vi "Telegram-Example.vi"() -> ()   [LabVIEW 2015]
doc: "Created IvanLis by LabVIEW Portal\nProfile: http://labviewportal.org/memberlist.php?mode=viewprofile&u=987\neMail: IvanLisanov@gMail.com\nTelegram: https://t.me/IvanLis"
uses:
  TypeDef/Client Command TypeDef.ctl
  TypeDef/Command Enum TypeDef.ctl
  Telegram Library/Telegram Class/Telegram Class.lvclass
  <vilib>/event_ctls.llb/usereventprio.ctl
  JSON Library/TypeDef/Message Text Out.ctl
  Telegram Library/TypeDef/TDLib Parameters.ctl
  JSON Library/JSON Library.lvlib
  Telegram Library/Telegram Library.lvlib
panel:
  in  "Message's":string
  in  "Message Out":string
  in  "Tab Control":enum32{"Chat's", "User's"}(tab)
  in  "Chat's":i32(listbox)
  in  "User's":i32(listbox)
  in  "Send Message":bool
  out "ConnectionState":string
  out "JSON":string
  out "Client ID":i32
  out "error":errorcluster
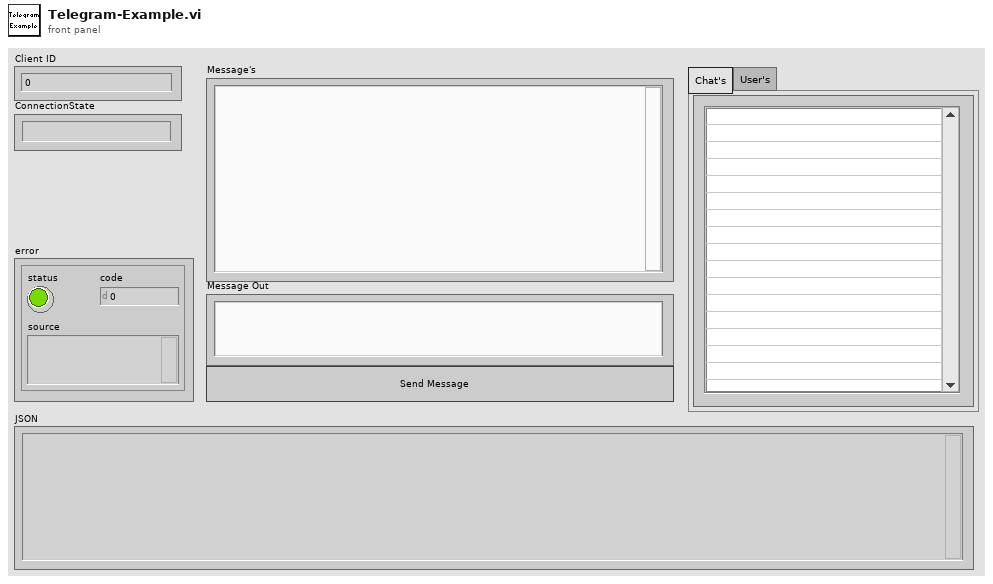
[diagram p1: front panel]
types:
  T1 = typedef "Client Command TypeDef.ctl" = cluster{"Command":T2, "Data":variant}
  T2 = typedef "Command Enum TypeDef.ctl" = enum16{"empty", "ClearControl", "Client Initialize", "Client Destroy", "Client Create", "Log Verbosity", "Test Execute", "Client Start", "Client Receive", "send_setTdlibParameters", "send_checkDatabaseEncryptionKey", "send_authorizationStateWaitPhoneNumber", "send_authorizationStateWaitCode", "send_getChats", "send_getChatHistory", "connectionState", "SendMessage", "Select Chat", "Select User"}
  T3 = typedef "usereventprio.ctl" = enum32{"high priority", "normal priority"}
  T4 = cluster{"@type":string, "new_verbosity_level":i32}
  T5 = cluster{"@type":string, "text":string, "@extra":string}
  T6 = typedef "JSON Library.lvlib/Message Text Out.ctl" = cluster{"@type":string, "chat_id":i64, "input_message_content":cluster{"@type":string, "text":cluster{"@type":string, "text":string}}}
  T7 = typedef "Telegram Library.lvlib/TDLib Parameters.ctl" = cluster{"database_directory":string, "use_file_database":bool, "use_chat_info_database":bool, "use_message_database":bool, "use_secret_chats":bool, "api_id":i32, "api_hash":string, "system_language_code":string, "device_model":string, "application_version":string, "enable_storage_optimizer":bool}
  T8 = cluster{"@type":string, "chat_id":i64, "from_message_id":i64, "limit":i32, "onlyLocal":bool}
  T9 = typedef "Telegram Library.lvlib/Telegram State.ctl" = enum16{"empty", "ok", "authorizationStateClosed", "authorizationStateWaitTdlibParameters", "authorizationStateWaitEncryptionKey", "authorizationStateWaitPhoneNumber", "authorizationStateWaitCode", "connectionStateWaitingForNetwork", "connectionStateConnectingToProxy", "connectionStateUpdating", "connectionStateConnecting", "connectionStateReady", "updateUser_user", "updateNewChat_chat", "updateNewMessage_Text", "updateChatLastMessage_Text", "updateDeleteMessages", "updateChatPosition", "ChatHistoryMessages_Text"}
  T10 = typedef "Telegram Library.lvlib/Chat.ctl" = cluster{"id":i64, "position":i64, "title":string}
  T11 = typedef "Telegram Library.lvlib/User.ctl" = cluster{"id":i64, "phone_number":string, "username":string, "last_name":string, "first_name":string}
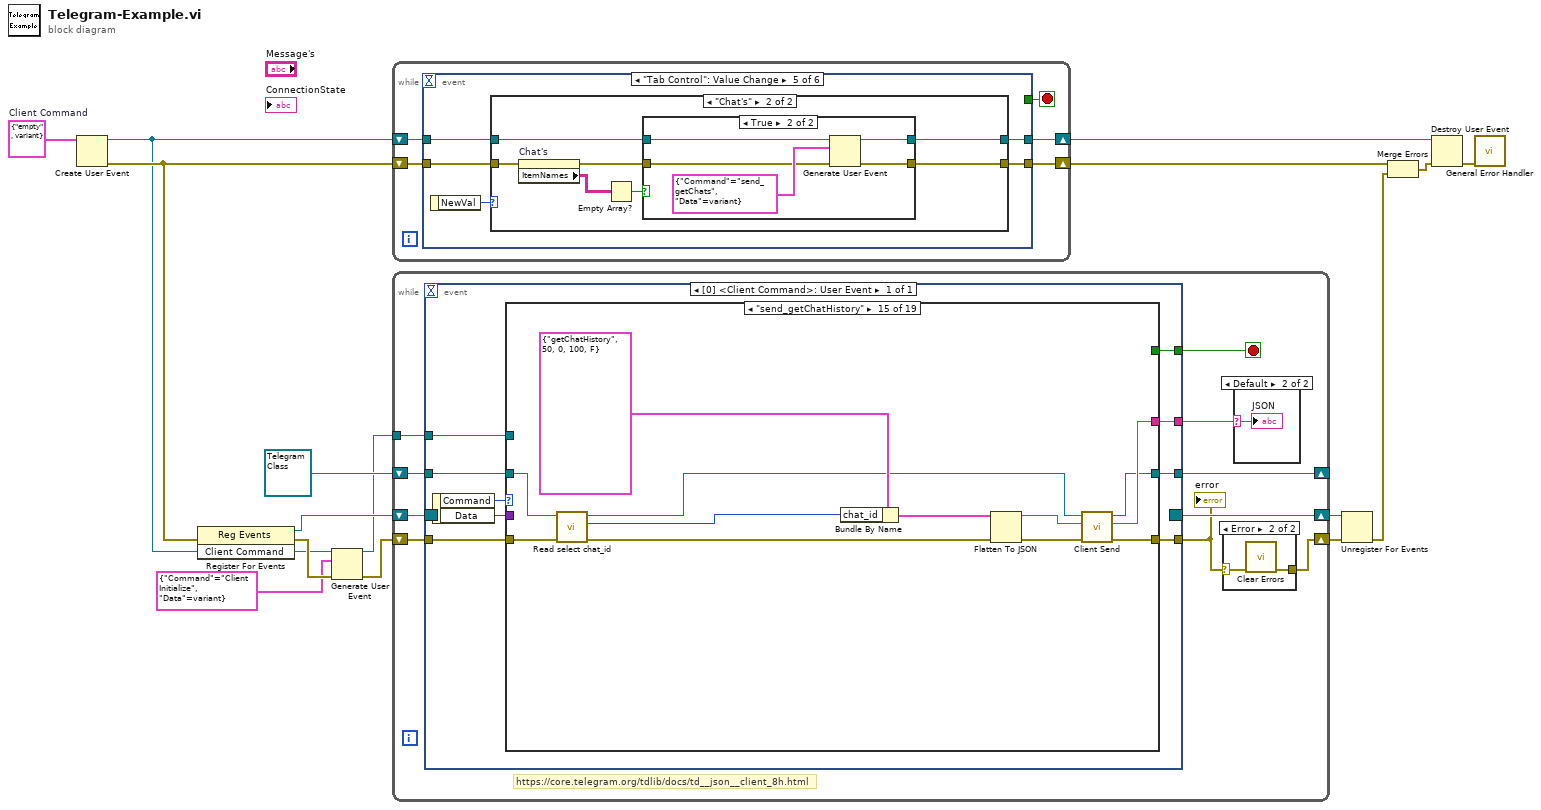
[diagram p0: block diagram]
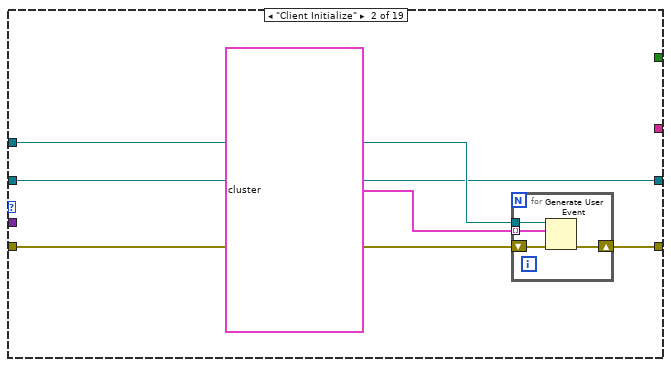
[diagram p5: hidden frame]
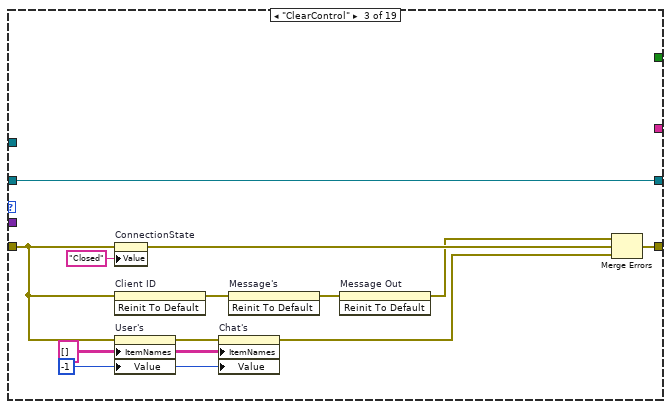
[diagram p6: hidden frame]
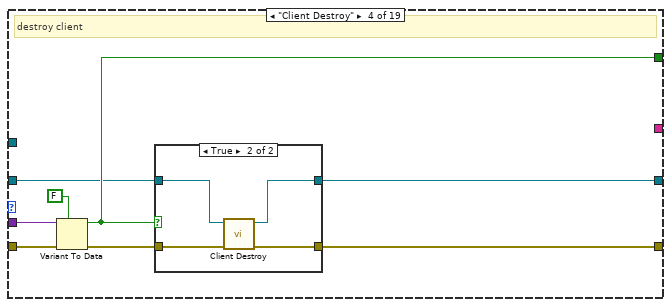
[diagram p7: hidden frame]
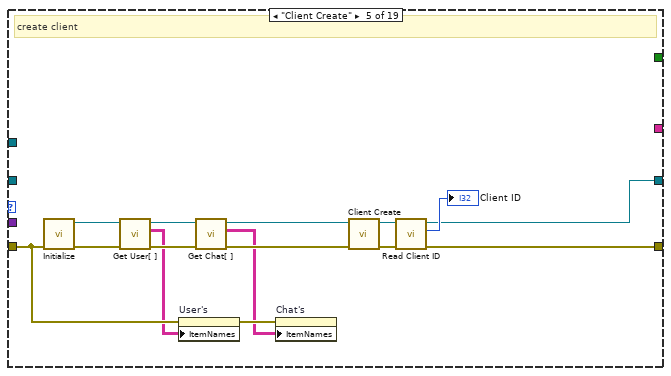
[diagram p9: hidden frame]
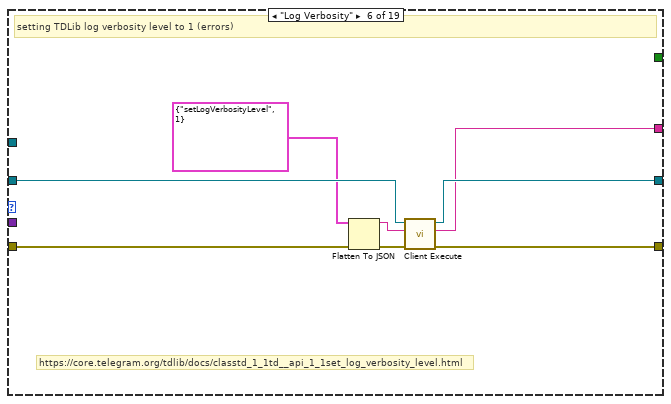
[diagram p10: hidden frame]
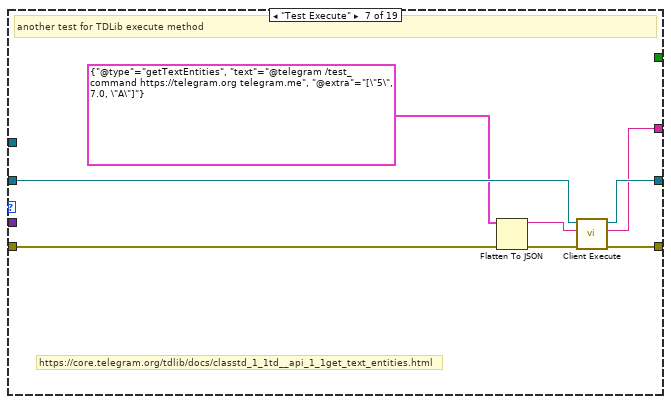
[diagram p11: hidden frame]
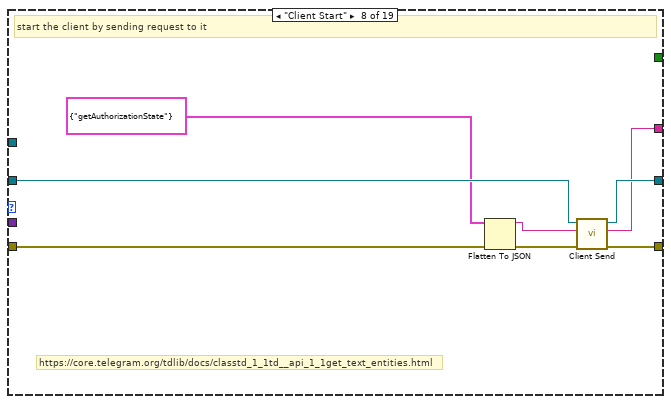
[diagram p12: hidden frame]
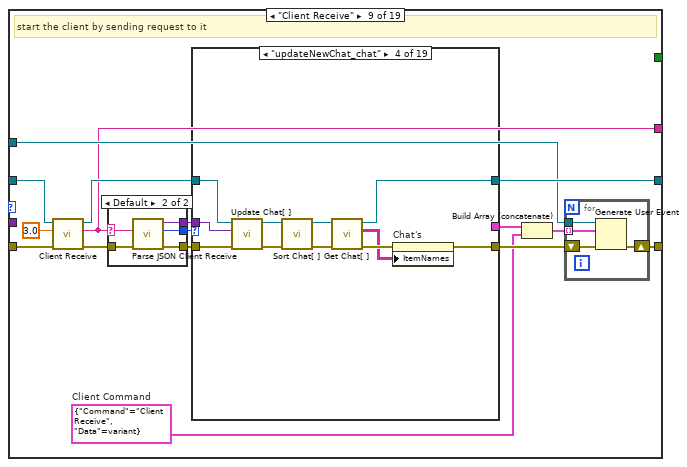
[diagram p13: hidden frame]
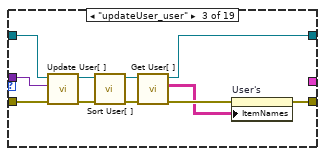
[diagram p17: hidden frame]
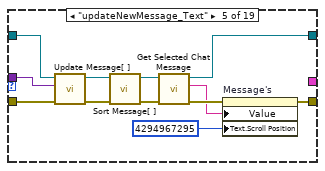
[diagram p18: hidden frame]
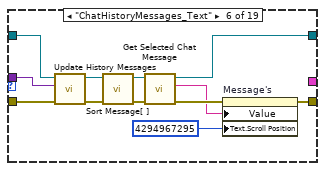
[diagram p19: hidden frame]
diagram:
  w15 = T1 {"Command"=enum."empty", "Data"=variant}  # Client Command
  n1 = Create User Event(user event datatype=w15) -> (user event=w3:refnum<user-event>, error out=w14:errorcluster)  [unwired: 1 in]
  n2 = register-events(error in=w14, w3) -> (reference out=w13:refnum<event-registration>, error out=w5:errorcluster)  [unwired: 1 in]
  n3 = Generate User Event(user event=w3, event data cluster=T1 {"Command"=enum."Client Initialize", "Data"=variant} ("event data"), error in=w5) -> (user event out=w2:refnum<user-event>, error out=w6:errorcluster)  [unwired: 1 in]
  n4 = while {
    shift-right: [w18] -> w10
    shift-left: w3 -> [w20]
    shift-right: [w17] -> w16
    shift-left: w14 -> [w19]
    stop <- w21 stop-if-true
    n5 = event shown="[4] \"Tab Control\": Value Change" {
      selector: _ -> [_ _ _ _ _ _]
      dyn-events: _ -> [_ _ _ _ _ _]
      timeout: _ -> [_ _ _ _ _ _]
      tunnel: [_ _ _ _ _ w71] -> w21
      tunnel: w20 -> [w26 w33 w40 w45 w50 w76]
      tunnel: w19 -> [w25 w32 w39 w44 w49 w75]
      tunnel: [w28 w35 w42 w47 w52 w78] -> w18
      tunnel: [w27 w34 w41 w46 w51 w77] -> w17
      event "Send Message": Value Change {
        n6 = event-data() -> ()  [unwired: 1 in, 1 out]
        n7 = Bundle By Name(cluster=T1 {"Command"=enum."SendMessage", "Data"=variant} ("event data"), "Data"="Message Out") -> (w23:T1)
        n8 = Generate User Event(user event=w26, event data cluster=w23, error in=w25) -> (user event out=w28:refnum<user-event>, error out=w27:errorcluster)  [unwired: 1 in]
      }
      event "Chat's": Value Change {
        n9 = event-data() -> ("NewVal"=w29:i32)  [unwired: 1 in]
        n10 = Bundle By Name(cluster=T1 {"Command"=enum."Select Chat", "Data"=variant} ("event data"), "Data"=w29) -> (w30:T1)
        n11 = Generate User Event(user event=w33, event data cluster=w30, error in=w32) -> (user event out=w35:refnum<user-event>, error out=w34:errorcluster)  [unwired: 1 in]
      }
      event "User's": Value Change {
        n12 = event-data() -> ("NewVal"=w36:i32)  [unwired: 1 in]
        n13 = Bundle By Name(cluster=T1 {"Command"=enum."Select User", "Data"=variant} ("event data"), "Data"=w36) -> (w37:T1)
        n14 = Generate User Event(user event=w40, event data cluster=w37, error in=w39) -> (user event out=w42:refnum<user-event>, error out=w41:errorcluster)  [unwired: 1 in]
      }
      event "Chat's": Double Click {
        n15 = event-data() -> ()  [unwired: 1 in, 4 out]
        n16 = Generate User Event(user event=w45, event data cluster=T1 {"Command"=enum."send_getChatHistory", "Data"=variant} ("event data"), error in=w44) -> (user event out=w47:refnum<user-event>, error out=w46:errorcluster)  [unwired: 1 in]
      }
      event "Tab Control": Value Change {
        n17 = event-data() -> ("NewVal"=w48:enum32{"Chat's", "User's"})  [unwired: 1 in]
        n18 = case shown="\"Chat's\"" w48 {
          tunnel: [w54 w61] -> w52
          tunnel: [w53 w60] -> w51
          tunnel: w50 -> [w54 w59]
          tunnel: w49 -> [w53 w58]
          frame Default {
          }
          frame "Chat's" {
            n19 = property on="Chat's" class="MCListbox (strict)"(error in=w58) -> (error out=w57:errorcluster, "ItemNames"=w56:string[][])  [unwired: 1 in, 1 out]
            n20 = Empty Array?(array=w56) -> (empty?=w55:bool)
            n21 = case shown="True" w55 {
              tunnel: [w63 w68] -> w61
              tunnel: [w62 w67] -> w60
              tunnel: w59 -> [w63 w66]
              tunnel: w57 -> [w62 w64]
              frame False {
              }
              frame True {
                n22 = Generate User Event(user event=w66, event data cluster=T1 {"Command"=enum."send_getChats", "Data"=variant} ("event data"), error in=w64) -> (user event out=w68:refnum<user-event>, error out=w67:errorcluster)  [unwired: 1 in]
              }
            }
          }
        }
      }
      event Panel Close? {
        w71 = TRUE
        n23 = event-data() -> ()  [unwired: 1 in, 1 out]
        n24 = Bundle By Name(cluster=T1 {"Command"=enum."Client Destroy", "Data"=variant} ("event data"), "Data"=w71) -> (w72:T1)
        n25 = Build Array(T1 {"Command"=enum."ClearControl", "Data"=variant} ("event data"), w72) -> (w70:T1[])
        n26 = for {
          tunnel: usereventprio."high priority" ("priority (normal)") -> [w80]
          tunnel: w70 -> [w79] mode=indexing
          shift-right: [w84] -> w78
          shift-left: w76 -> [w82]
          shift-right: [w83] -> w77
          shift-left: w75 -> [w81]
          n27 = Generate User Event(priority (normal)=w80, user event=w82, event data cluster=w79, error in=w81) -> (user event out=w84:refnum<user-event>, error out=w83:errorcluster)
        }
        n28 = event-data("Discard?"=w71) -> ()  [unwired: 1 in, 1 out]
      }
    }
  }
  n29 = while {
    shift-right: [w91] -> w12
    shift-left: w13 -> [w93]
    shift-right: [w85] -> w11
    shift-left: w6 -> [w92]
    tunnel: w2 -> [w88]
    shift-right: [w90] -> _
    shift-left: refnum<class "Telegram Class.lvclass"> refnum ("Telegram Class out") -> [w89]
    stop <- w94 stop-if-true
    # "https://core.telegram.org/tdlib/docs/td__json__client_8h.html"
    n30 = event shown="[0] <Client Command>: User Event" {
      selector: w93 -> [_]
      dyn-events: [_] -> w91
      timeout: _ -> [_]
      tunnel: [w103] -> w94
      tunnel: w92 -> [w107]
      tunnel: [w104] -> w86
      tunnel: [w102] -> w90
      tunnel: w89 -> [w101]
      tunnel: [w100] -> w87
      tunnel: w88 -> [w99]
      event User Event {
        n31 = event-data() -> ("Command"=w106:T2, "Data"=w105:variant)  [unwired: 1 in]
        n32 = case shown="\"send_getChatHistory\"" w106 {
          tunnel: w107 -> [w109 w110 w123 w138 w147 w162 w170 w177 w199 w336 w360 w370 w378 w386 w397 w409 w419 w456 w471]
          tunnel: w105 -> [_ _ _ w137 _ _ _ _ _ w335 w361 _ _ _ _ _ _ w455 w470]
          tunnel: [w109 w114 w122 w133 w149 w167 w175 w183 w190 w345 w362 w375 w383 w391 w403 w415 w424 w439 w472] -> w104
          tunnel: [_ _ _ w135 _ _ _ _ _ _ _ _ _ _ _ _ _ _ _] -> w103
          tunnel: [w108 w111 w127 w132 w150 w165 w173 w181 w193 w346 w363 w373 w381 w389 w401 w413 w422 w444 w473] -> w102
          tunnel: w101 -> [w108 w111 w127 w131 _ w166 w174 w182 w198 w340 w363 w369 w376 w384 w396 w405 w420 w457 w474]
          tunnel: [_ _ _ _ _ w164 w172 w180 w187 w344 _ w374 w382 w390 w402 w414 w423 _ _] -> w100
          tunnel: w99 -> [_ w113 _ _ _ _ _ _ w188 _ _ _ _ _ _ _ _ w438 _]
          frame "empty" {
          }
          frame "Client Initialize" {
            n33 = for {
              shift-right: [w117] -> w114
              shift-left: w110 -> [w118]
              tunnel: w113 -> [w116]
              tunnel: T1[] [{"Command"=enum."ClearControl", "Data"=variant}, {"Command"=enum."Client Create", "Data"=variant}, {"Command"=enum."Log Verbosity", "Data"=variant}, {"Command"=enum."Test Execute", "Data"=variant}, {"Command"=enum."Client Start", "Data"=variant}, {"Command"=enum."Client Receive", "Data"=variant}] -> [w115] mode=indexing
              n34 = Generate User Event(user event=w116, event data cluster=w115, error in=w118) -> (error out=w117:errorcluster)  [unwired: 1 in, 1 out]
            }
          }
          frame "ClearControl" {
            w126 = string[][] [] ("Item Names")
            w129 = -1 ("Focus Row")
            n35 = property on="ConnectionState" class="Str"(error in=w123, "Value"="Closed" ("ConnectionState")) -> (error out=w121:errorcluster)  [unwired: 1 in, 1 out]
            n36 = invoke on="Client ID" class="DigNum (strict)" method="Reinit To Default"(error in=w123) -> (error out=w124:errorcluster)  [unwired: 2 in, 2 out]
            n37 = property on="User's" class="MCListbox (strict)"(error in=w123, "ItemNames"=w126, "Value"=w129) -> (error out=w128:errorcluster)  [unwired: 1 in, 1 out]
            n38 = property on="Chat's" class="MCListbox (strict)"(error in=w128, "ItemNames"=w126, "Value"=w129) -> (error out=w119:errorcluster)  [unwired: 1 in, 1 out]
            n39 = invoke on="Message's" class="Str" method="Reinit To Default"(error in=w124) -> (error out=w125:errorcluster)  [unwired: 2 in, 2 out]
            n40 = invoke on="Message Out" class="Str" method="Reinit To Default"(error in=w125) -> (error out=w120:errorcluster)  [unwired: 2 in, 2 out]
            n41 = Merge Errors(w120, w121, w119) -> (w122:errorcluster)
          }
          frame "Client Destroy" {
            # "destroy client"
            n42 = Variant To Data(error in=w138, type=FALSE, Variant=w137) -> (data=w135:bool, error out=w134:errorcluster)
            n43 = case shown="True" w135 {
              tunnel: w134 -> [w139 w144]
              tunnel: [w139 w141] -> w133
              tunnel: [w140 w142] -> w132
              tunnel: w131 -> [w140 w143]
              frame False {
              }
              frame True {
                n44 = call-dynamic "Client Destroy.vi"("error in (no error)"=w144, "Telegram Class in"=w143) -> ("error out"=w141:errorcluster, "Telegram Class out"=w142:refnum<class "Telegram Class.lvclass">)  [unwired: 8 in]
              }
            }
          }
          frame "Client Create" {
            # "create client"
            n45 = call "Initialize.vi"("error in (no error)"=w147) -> ("error out"=w154:errorcluster, "Telegram Class out"=w155:refnum<class "Telegram Class.lvclass">)  [unwired: 9 in]
            n46 = call-dynamic "Get User[ ].vi"("error in (no error)"=w154, "Telegram Class in"=w155) -> ("error out"=w153:errorcluster, "User[ ]"=w146:string[][], "Telegram Class out"=w156:refnum<class "Telegram Class.lvclass">)  [unwired: 7 in]
            n47 = property on="User's" class="MCListbox (strict)"(error in=w147, "ItemNames"=w146) -> (error out=w148:errorcluster)  [unwired: 1 in, 1 out]
            n48 = call-dynamic "Get Chat[ ].vi"("error in (no error)"=w153, "Telegram Class in"=w156) -> ("error out"=w152:errorcluster, "Chat[ ]"=w145:string[][], "Telegram Class out"=w151:refnum<class "Telegram Class.lvclass">)  [unwired: 7 in]
            n49 = property on="Chat's" class="MCListbox (strict)"(error in=w148, "ItemNames"=w145) -> ()  [unwired: 1 in, 2 out]
            n50 = call-dynamic "Client Create.vi"("error in (no error)"=w152, "Telegram Class in"=w151) -> ("error out"=w159:errorcluster, "Telegram Class out"=w158:refnum<class "Telegram Class.lvclass">)  [unwired: 8 in]
            n51 = call-dynamic "Read Client ID.vi"("error in (no error)"=w159, "Telegram Class in"=w158) -> ("error out"=w149:errorcluster, "Client ID"=→"Client ID":i32, "Telegram Class out"=w150:refnum<class "Telegram Class.lvclass">)  [unwired: 7 in]
          }
          frame "Log Verbosity" {
            # "https://core.telegram.org/tdlib/docs/classtd_1_1td__api_1_1set_log_verbosity_level.html"
            # "setting TDLib log verbosity level to 1 (errors)"
            n52 = Flatten To JSON(anything=T4 {"@type"="setLogVerbosityLevel", "new_verbosity_level"=1}, error in (no error)=w162) -> (JSON string=w161:string, 11:w163:errorcluster)  [unwired: 1 in]
            n53 = call-dynamic "Client Execute.vi"("error in (no error)"=w163, "JSON (UTF-8) String In"=w161, "Telegram Class in"=w166) -> ("error out"=w167:errorcluster, "UTF-8 String Out"=w164:string, "Telegram Class out"=w165:refnum<class "Telegram Class.lvclass">)  [unwired: 6 in]
          }
          frame "Test Execute" {
            # "https://core.telegram.org/tdlib/docs/classtd_1_1td__api_1_1get_text_entities.html"
            # "another test for TDLib execute method"
            n54 = Flatten To JSON(anything=T5 {"@type"="getTextEntities", "text"="@telegram /test_command https://telegram.org telegram.me", "@extra"="[\"5\", 7.0, \"A\"]"}, error in (no error)=w170) -> (JSON string=w169:string, 11:w171:errorcluster)  [unwired: 1 in]
            n55 = call-dynamic "Client Execute.vi"("error in (no error)"=w171, "JSON (UTF-8) String In"=w169, "Telegram Class in"=w174) -> ("error out"=w175:errorcluster, "UTF-8 String Out"=w172:string, "Telegram Class out"=w173:refnum<class "Telegram Class.lvclass">)  [unwired: 6 in]
          }
          frame "Client Start" {
            # "https://core.telegram.org/tdlib/docs/classtd_1_1td__api_1_1get_text_entities.html"
            # "start the client by sending request to it"
            n56 = Flatten To JSON(anything=cluster{"@type":string} {"@type"="getAuthorizationState"} ("Message"), error in (no error)=w177) -> (JSON string=w179:string, 11:w178:errorcluster)  [unwired: 1 in]
            n57 = call-dynamic "Client Send.vi"("error in (no error)"=w178, "JSON (UTF-8) String In"=w179, "Telegram Class in"=w182) -> ("error out"=w183:errorcluster, "UTF-8 String Out"=w180:string, "Telegram Class out"=w181:refnum<class "Telegram Class.lvclass">)  [unwired: 6 in]
          }
          frame "Client Receive" {
            w184 = T1 {"Command"=enum."Client Receive", "Data"=variant}  # Client Command
            # "start the client by sending request to it"
            n58 = call-dynamic "Client Receive.vi"("error in (no error)"=w199, "Timeout"=3.0, "Telegram Class in"=w198) -> ("error out"=w196:errorcluster, "UTF-8 String Out"=w187:string, "Telegram Class out"=w192:refnum<class "Telegram Class.lvclass">)  [unwired: 6 in]
            n59 = case shown="Default" w187 {
              selector: w187 -> [_ w202]
              tunnel: w196 -> [w200 w205]
              tunnel: [_ w204] -> w195
              tunnel: [w200 w203] -> w194
              tunnel: [_ w201] -> w186
              frame "" {
              }
              frame Default {
                n60 = call "Parse JSON Client Receive.vi"("error in (no error)"=w205, "JSON (UTF-8) String"=w202) -> ("error out"=w203:errorcluster, "Telegram State"=w204:T9, "Message"=w201:variant)  [unwired: 7 in]
              }
            }
            n61 = case shown="\"updateNewChat_chat\"" w195 {
              tunnel: w194 -> [w210 w212 w224 w235 w247 w259 w260 w272 w277 w283 w286 w289 w292 w295 w301 w307 w313 w319 w326]
              tunnel: [w211 w213 w220 w231 w243 w255 w261 w267 w274 w284 w287 w290 w293 w296 w302 w308 w314 w320 w327] -> w193
              tunnel: w192 -> [w211 w213 w223 w234 w246 w258 w261 w271 w275 w284 w287 w290 w293 w296 w302 w308 w314 w320 w327]
              tunnel: [w210 w212 w221 w232 w244 w256 w260 w266 w276 w283 w286 w289 w292 w295 w301 w307 w313 w319 w326] -> w191
              tunnel: [_ _ _ _ _ _ _ _ _ w281 w285 w288 w291 w294 w299 w305 w311 w317 w324] -> w189
              tunnel: w186 -> [_ _ w222 w233 w245 w257 _ w270 w273 _ _ _ _ _ _ _ _ _ _]
              frame "empty" {
              }
              frame "ok" {
              }
              frame "updateUser_user" {
                n62 = call-dynamic "Update User[ ].vi"("error in (no error)"=w224, "Message"=w222, "Telegram Class in"=w223) -> ("error out"=w216:errorcluster, "Telegram Class out"=w217:refnum<class "Telegram Class.lvclass">)  [unwired: 7 in]
                n63 = call-dynamic "Sort User[ ].vi"("error in (no error)"=w216, "Telegram Class in"=w217) -> ("error out"=w214:errorcluster, "Telegram Class out"=w215:refnum<class "Telegram Class.lvclass">)  [unwired: 8 in]
                n64 = call-dynamic "Get User[ ].vi"("error in (no error)"=w214, "Telegram Class in"=w215) -> ("error out"=w219:errorcluster, "User[ ]"=w218:string[][], "Telegram Class out"=w220:refnum<class "Telegram Class.lvclass">)  [unwired: 7 in]
                n65 = property on="User's" class="MCListbox (strict)"(error in=w219, "ItemNames"=w218) -> (error out=w221:errorcluster)  [unwired: 1 in, 1 out]
              }
              frame "updateNewChat_chat" {
                n66 = call-dynamic "Update Chat[ ].vi"("error in (no error)"=w235, "Message"=w233, "Telegram Class in"=w234) -> ("error out"=w228:errorcluster, "Telegram Class out"=w225:refnum<class "Telegram Class.lvclass">)  [unwired: 7 in]
                n67 = call-dynamic "Sort Chat[ ].vi"("error in (no error)"=w228, "Telegram Class in"=w225) -> ("error out"=w227:errorcluster, "Telegram Class out"=w226:refnum<class "Telegram Class.lvclass">)  [unwired: 8 in]
                n68 = call-dynamic "Get Chat[ ].vi"("error in (no error)"=w227, "Telegram Class in"=w226) -> ("error out"=w230:errorcluster, "Chat[ ]"=w229:string[][], "Telegram Class out"=w231:refnum<class "Telegram Class.lvclass">)  [unwired: 7 in]
                n69 = property on="Chat's" class="MCListbox (strict)"(error in=w230, "ItemNames"=w229) -> (error out=w232:errorcluster)  [unwired: 1 in, 1 out]
              }
              frame "updateNewMessage_Text" {
                n70 = call-dynamic "Update Message[ ].vi"("error in (no error)"=w247, "Message"=w245, "Telegram Class in"=w246) -> ("error out"=w238:errorcluster, "Telegram Class out"=w239:refnum<class "Telegram Class.lvclass">)  [unwired: 7 in]
                n71 = call-dynamic "Sort Message[ ].vi"("error in (no error)"=w238, "Telegram Class in"=w239) -> ("error out"=w236:errorcluster, "Telegram Class out"=w237:refnum<class "Telegram Class.lvclass">)  [unwired: 8 in]
                n72 = call-dynamic "Get Selected Chat Message.vi"("error in (no error)"=w236, "Telegram Class in"=w237) -> ("error out"=w242:errorcluster, "Message's"=w241:string, "Telegram Class out"=w243:refnum<class "Telegram Class.lvclass">)  [unwired: 7 in]
                n73 = property on="Message's" class="Str"(error in=w242, "Value"=w241, "Text.Scroll Position"=u32 4294967295) -> (error out=w244:errorcluster)  [unwired: 1 in, 1 out]
              }
              frame "ChatHistoryMessages_Text" {
                n74 = call-dynamic "Update History Messages.vi"("error in (no error)"=w259, "Message"=w257, "Telegram Class in"=w258) -> ("error out"=w248:errorcluster, "Telegram Class out"=w251:refnum<class "Telegram Class.lvclass">)  [unwired: 7 in]
                n75 = call-dynamic "Sort Message[ ].vi"("error in (no error)"=w248, "Telegram Class in"=w251) -> ("error out"=w249:errorcluster, "Telegram Class out"=w250:refnum<class "Telegram Class.lvclass">)  [unwired: 8 in]
                n76 = call-dynamic "Get Selected Chat Message.vi"("error in (no error)"=w249, "Telegram Class in"=w250) -> ("error out"=w254:errorcluster, "Message's"=w253:string, "Telegram Class out"=w255:refnum<class "Telegram Class.lvclass">)  [unwired: 7 in]
                n77 = property on="Message's" class="Str"(error in=w254, "Value"=w253, "Text.Scroll Position"=u32 4294967295) -> (error out=w256:errorcluster)  [unwired: 1 in, 1 out]
              }
              frame "updateChatLastMessage_Text" {
              }
              frame "updateChatPosition" {
                n78 = call-dynamic "Update Chat Position.vi"("error in (no error)"=w272, "Message"=w270, "Telegram Class in"=w271) -> ("error out"=w265:errorcluster, "Telegram Class out"=w269:refnum<class "Telegram Class.lvclass">)  [unwired: 7 in]
                n79 = call-dynamic "Sort Chat[ ].vi"("error in (no error)"=w265, "Telegram Class in"=w269) -> ("error out"=w264:errorcluster, "Telegram Class out"=w268:refnum<class "Telegram Class.lvclass">)  [unwired: 8 in]
                n80 = call-dynamic "Get Chat[ ].vi"("error in (no error)"=w264, "Telegram Class in"=w268) -> ("error out"=w263:errorcluster, "Chat[ ]"=w262:string[][], "Telegram Class out"=w267:refnum<class "Telegram Class.lvclass">)  [unwired: 7 in]
                n81 = property on="Chat's" class="MCListbox (strict)"(error in=w263, "ItemNames"=w262) -> (error out=w266:errorcluster)  [unwired: 1 in, 1 out]
              }
              frame "updateDeleteMessages" {
                n82 = call-dynamic "Delete Messages.vi"("error in (no error)"=w277, "Message"=w273, "Telegram Class in"=w275) -> ("error out"=w276:errorcluster, "Telegram Class out"=w274:refnum<class "Telegram Class.lvclass">)  [unwired: 7 in]
              }
              frame "authorizationStateClosed" {
                # "if client is closed, we need to destroy it and create new client"
                n83 = Bundle By Name(cluster=T1 {"Command"=enum."connectionState", "Data"=variant} ("event data"), "Data"="Closed") -> (w279:T1)
                n84 = Build Array (concatenate)(w279, T1[] [{"Command"=enum."Client Destroy", "Data"=variant}, {"Command"=enum."Client Create", "Data"=variant}, {"Command"=enum."Log Verbosity", "Data"=variant}, {"Command"=enum."Test Execute", "Data"=variant}, {"Command"=enum."Client Start", "Data"=variant}]) -> (w281:T1[])
              }
              frame "authorizationStateWaitTdlibParameters" {
                w285 = T1[] [{"Command"=enum."send_setTdlibParameters", "Data"=variant}]  # Client Command's
                # "set TDLib parameters\nyou MUST obtain your own api_id and api_hash at \nhttps://my.telegram.org\nand use them in the setTdlibParameters call"
              }
              frame "authorizationStateWaitEncryptionKey" {
                w288 = T1[] [{"Command"=enum."send_checkDatabaseEncryptionKey", "Data"=variant}]  # Client Command's
                # "set an encryption key for database to let know TDLib how to open the database"
              }
              frame "authorizationStateWaitPhoneNumber" {
                w291 = T1[] [{"Command"=enum."send_authorizationStateWaitPhoneNumber", "Data"=variant}]  # Client Command's
                # "enter phone number to log in"
              }
              frame "authorizationStateWaitCode" {
                w294 = T1[] [{"Command"=enum."send_authorizationStateWaitCode", "Data"=variant}]  # Client Command's
                # "wait for authorization code"
              }
              frame "connectionStateConnecting" {
                # "updateConnectionState"
                n85 = Bundle By Name(cluster=T1 {"Command"=enum."connectionState", "Data"=variant} ("Client Command"), "Data"="Connecting") -> (w298:T1)
                n86 = Build Array(w298) -> (w299:T1[])
              }
              frame "connectionStateWaitingForNetwork" {
                # "updateConnectionState"
                n87 = Bundle By Name(cluster=T1 {"Command"=enum."connectionState", "Data"=variant} ("Client Command"), "Data"="WaitingForNetwork") -> (w304:T1)
                n88 = Build Array(w304) -> (w305:T1[])
              }
              frame "connectionStateConnectingToProxy" {
                # "updateConnectionState"
                n89 = Bundle By Name(cluster=T1 {"Command"=enum."connectionState", "Data"=variant} ("Client Command"), "Data"="ConnectingToProxy") -> (w310:T1)
                n90 = Build Array(w310) -> (w311:T1[])
              }
              frame "connectionStateUpdating" {
                # "updateConnectionState"
                n91 = Bundle By Name(cluster=T1 {"Command"=enum."connectionState", "Data"=variant} ("Client Command"), "Data"="Updating") -> (w316:T1)
                n92 = Build Array(w316) -> (w317:T1[])
              }
              frame "connectionStateReady" {
                w325 = T1[] [{"Command"=enum."send_getChats", "Data"=variant}]  # Client Command's
                # "updateConnectionState"
                n93 = Bundle By Name(cluster=T1 {"Command"=enum."connectionState", "Data"=variant} ("Client Command"), "Data"="Ready") -> (w322:T1)
                n94 = Build Array (concatenate)(w322, w325) -> (w324:T1[])
              }
            }
            n95 = Build Array (concatenate)(w189, w184) -> (w185:T1[])
            n96 = for {
              shift-right: [w208] -> w190
              shift-left: w191 -> [w209]
              tunnel: w185 -> [w207] mode=indexing
              tunnel: w188 -> [w206]
              n97 = Generate User Event(user event=w206, event data cluster=w207, error in=w209) -> (error out=w208:errorcluster)  [unwired: 1 in, 1 out]
            }
          }
          frame "SendMessage" {
            n98 = Variant To Data(error in=w336, type="", Variant=w335) -> (data=w332:string, error out=w334:errorcluster)
            n99 = case shown="\"Chat's\", Default" "Tab Control" {
              tunnel: w340 -> [w350 w355]
              tunnel: w334 -> [w351 w356]
              tunnel: [w348 w354] -> w339
              tunnel: [w349 w352] -> w331
              tunnel: [w347 w353] -> w328
              frame "Chat's", Default {
                n100 = call-dynamic "Read select chat_id.vi"("error in (no error)"=w351, "Telegram Class in"=w350) -> ("error out"=w349:errorcluster, "select chat_id"=w347:i64, "Telegram Class out"=w348:refnum<class "Telegram Class.lvclass">)  [unwired: 7 in]
              }
              frame "User's" {
                n101 = call-dynamic "Read select user_id.vi"("error in (no error)"=w356, "Telegram Class in"=w355) -> ("error out"=w352:errorcluster, "select user_id"=w353:i64, "Telegram Class out"=w354:refnum<class "Telegram Class.lvclass">)  [unwired: 7 in]
              }
            }
            n102 = Bundle By Name(cluster=T6 {"@type"="sendMessage", "chat_id"=-662715306, "input_message_content"={"@type"="inputMessageText", "text"={"@type"="formattedText", "text"="Test From LabVIEW Bot\nÒåñò áîòà ËàáÂüþ"}}} ("Message"), "chat_id"=w328, "input_message_content.text.text"=w332) -> (w338:T6)
            n103 = property on="Message Out" class="Str"(error in=w331, "Value"="" ("Message Out")) -> (error out=w330:errorcluster)  [unwired: 1 in, 1 out]
            n104 = Flatten To JSON(anything=w338, error in (no error)=w330) -> (JSON string=w342:string, 11:w343:errorcluster)  [unwired: 1 in]
            n105 = call-dynamic "Client Send.vi"("error in (no error)"=w343, "JSON (UTF-8) String In"=w342, "Telegram Class in"=w339) -> ("error out"=w345:errorcluster, "UTF-8 String Out"=w344:string, "Telegram Class out"=w346:refnum<class "Telegram Class.lvclass">)  [unwired: 6 in]
          }
          frame "connectionState" {
            n106 = Variant To Data(error in=w360, type="" ("ConnectionState"), Variant=w361) -> (data=w357:string, error out=w358:errorcluster)
            n107 = property on="ConnectionState" class="Str"(error in=w358, "Value"=w357) -> (error out=w362:errorcluster)  [unwired: 1 in, 1 out]
          }
          frame "send_setTdlibParameters" {
            n108 = call-dynamic "Read parameters.vi"("error in (no error)"=w370, "Telegram Class in"=w369) -> ("error out"=w367:errorcluster, "parameters"=w364:T7, "Telegram Class out"=w368:refnum<class "Telegram Class.lvclass">)  [unwired: 7 in]
            n109 = Bundle By Name(cluster=cluster{"@type":string, "parameters":T7} {"@type"="setTdlibParameters", "parameters"={"database_directory"="tdlib", "use_file_database"=TRUE, "use_chat_info_database"=TRUE, "use_message_database"=TRUE, "use_secret_chats"=TRUE, "api_id"=0, "api_hash"="Desktop", "system_language_code"="0.1", "device_model"="Desktop", "application_version"="0.1", "enable_storage_optimizer"=TRUE}} ("setTdlibParameters"), "parameters"=w364) -> (w365:cluster{"@type":string, "parameters":T7})
            n110 = Flatten To JSON(anything=w365, error in (no error)=w367) -> (JSON string=w372:string, 11:w371:errorcluster)  [unwired: 1 in]
            n111 = call-dynamic "Client Send.vi"("error in (no error)"=w371, "JSON (UTF-8) String In"=w372, "Telegram Class in"=w368) -> ("error out"=w375:errorcluster, "UTF-8 String Out"=w374:string, "Telegram Class out"=w373:refnum<class "Telegram Class.lvclass">)  [unwired: 6 in]
          }
          frame "send_checkDatabaseEncryptionKey" {
            n112 = Flatten To JSON(anything=cluster{"@type":string, "encryption_key":string} {"@type"="checkDatabaseEncryptionKey", "encryption_key"=""} ("Message"), error in (no error)=w378) -> (JSON string=w380:string, 11:w379:errorcluster)  [unwired: 1 in]
            n113 = call-dynamic "Client Send.vi"("error in (no error)"=w379, "JSON (UTF-8) String In"=w380, "Telegram Class in"=w376) -> ("error out"=w383:errorcluster, "UTF-8 String Out"=w382:string, "Telegram Class out"=w381:refnum<class "Telegram Class.lvclass">)  [unwired: 6 in]
          }
          frame "send_getChats" {
            n114 = Flatten To JSON(anything=cluster{"@type":string, "limit":i32} {"@type"="getChats", "limit"=2147483647} ("Message"), error in (no error)=w386) -> (JSON string=w388:string, 11:w387:errorcluster)  [unwired: 1 in]
            n115 = call-dynamic "Client Send.vi"("error in (no error)"=w387, "JSON (UTF-8) String In"=w388, "Telegram Class in"=w384) -> ("error out"=w391:errorcluster, "UTF-8 String Out"=w390:string, "Telegram Class out"=w389:refnum<class "Telegram Class.lvclass">)  [unwired: 6 in]
          }
          frame "send_getChatHistory" {
            n116 = call-dynamic "Read select chat_id.vi"("error in (no error)"=w397, "Telegram Class in"=w396) -> ("error out"=w394:errorcluster, "select chat_id"=w392:i64, "Telegram Class out"=w395:refnum<class "Telegram Class.lvclass">)  [unwired: 7 in]
            n117 = Bundle By Name(cluster=T8 {"@type"="getChatHistory", "chat_id"=50, "from_message_id"=0, "limit"=100, "onlyLocal"=FALSE} ("Message"), "chat_id"=w392) -> (w393:T8)
            n118 = Flatten To JSON(anything=w393, error in (no error)=w394) -> (JSON string=w400:string, 11:w399:errorcluster)  [unwired: 1 in]
            n119 = call-dynamic "Client Send.vi"("error in (no error)"=w399, "JSON (UTF-8) String In"=w400, "Telegram Class in"=w395) -> ("error out"=w403:errorcluster, "UTF-8 String Out"=w402:string, "Telegram Class out"=w401:refnum<class "Telegram Class.lvclass">)  [unwired: 6 in]
          }
          frame "send_authorizationStateWaitPhoneNumber" {
            n120 = call-dynamic "Read phone_number.vi"("error in (no error)"=w409, "Telegram Class in"=w405) -> ("error out"=w408:errorcluster, "phone_number"=w406:string, "Telegram Class out"=w404:refnum<class "Telegram Class.lvclass">)  [unwired: 7 in]
            n121 = Bundle By Name(cluster=cluster{"@type":string, "phone_number":string} {"@type"="setAuthenticationPhoneNumber", "phone_number"="7 920-281-13-41"} ("Message"), "phone_number"=w406) -> (w407:cluster{"@type":string, "phone_number":string})
            n122 = Flatten To JSON(anything=w407, error in (no error)=w408) -> (JSON string=w412:string, 11:w411:errorcluster)  [unwired: 1 in]
            n123 = call-dynamic "Client Send.vi"("error in (no error)"=w411, "JSON (UTF-8) String In"=w412, "Telegram Class in"=w404) -> ("error out"=w415:errorcluster, "UTF-8 String Out"=w414:string, "Telegram Class out"=w413:refnum<class "Telegram Class.lvclass">)  [unwired: 6 in]
          }
          frame "send_authorizationStateWaitCode" {
            n124 = call "Enter Authentication Code.vi"("error in (no error)"=w419) -> ("error out"=w418:errorcluster, "Cencel"=w416:bool, "Authentication Code"=w417:string)  [unwired: 8 in]
            n125 = case shown="False" w416 {
              tunnel: [w434 w435] -> w424
              tunnel: [w433 _] -> w423
              tunnel: [w432 w436] -> w422
              tunnel: cluster{"@type":string, "code":string} {"@type"="checkAuthenticationCode", "code"=""} ("Message") -> [w429 _]
              tunnel: w420 -> [w428 w436]
              tunnel: w418 -> [w426 w435]
              tunnel: w417 -> [w425 _]
              frame False {
                n126 = Bundle By Name(cluster=w429, "code"=w425) -> (w427:cluster{"@type":string, "code":string})
                n127 = Flatten To JSON(anything=w427, error in (no error)=w426) -> (JSON string=w431:string, 11:w430:errorcluster)  [unwired: 1 in]
                n128 = call-dynamic "Client Send.vi"("error in (no error)"=w430, "JSON (UTF-8) String In"=w431, "Telegram Class in"=w428) -> ("error out"=w434:errorcluster, "UTF-8 String Out"=w433:string, "Telegram Class out"=w432:refnum<class "Telegram Class.lvclass">)  [unwired: 6 in]
              }
              frame True {
              }
            }
          }
          frame "Select Chat" {
            n129 = Variant To Data(error in=w456, type=0 ("NewVal"), Variant=w455) -> (data=w452:i32, error out=w453:errorcluster)
            n130 = call-dynamic "Read Chat[ ].vi"("error in (no error)"=w453, "Telegram Class in"=w457) -> ("error out"=w448:errorcluster, "Chat[ ]"=w451:T10[], "Telegram Class out"=w449:refnum<class "Telegram Class.lvclass">)  [unwired: 7 in]
            n131 = Index Array(array=w451, index=w452) -> (element=w450:T10)
            n132 = Unbundle By Name(w450) -> ("id"=w447:i64)
            n133 = call-dynamic "Write select chat_id.vi"("error in (no error)"=w448, "select chat_id"=w447, "Telegram Class in"=w449) -> ("error out"=w446:errorcluster, "Telegram Class out"=w445:refnum<class "Telegram Class.lvclass">)  [unwired: 7 in]
            n134 = call-dynamic "Get Selected Chat Message.vi"("error in (no error)"=w446, "Telegram Class in"=w445) -> ("error out"=w443:errorcluster, "Message's"=w442:string, "Telegram Class out"=w444:refnum<class "Telegram Class.lvclass">)  [unwired: 7 in]
            n135 = property on="Message's" class="Str"(error in=w443, "Value"=w442, "Text.Scroll Position"=u32 4294967295) -> (error out=w440:errorcluster)  [unwired: 1 in, 1 out]
            n136 = for {
              tunnel: w438 -> [w459]
              tunnel: T1[] [{"Command"=enum."send_getChatHistory", "Data"=variant}, {"Command"=enum."send_getChatHistory", "Data"=variant}] ("event data") -> [w458] mode=indexing
              shift-right: [w460] -> w439
              shift-left: w440 -> [w461]
              n137 = Generate User Event(user event=w459, event data cluster=w458, error in=w461) -> (error out=w460:errorcluster)  [unwired: 1 in, 1 out]
            }
          }
          frame "Select User" {
            n138 = Variant To Data(error in=w471, type=0 ("NewVal"), Variant=w470) -> (data=w462:i32, error out=w468:errorcluster)
            n139 = call-dynamic "Read User[ ].vi"("error in (no error)"=w468, "Telegram Class in"=w474) -> ("error out"=w464:errorcluster, "User[ ]"=w467:T11[], "Telegram Class out"=w465:refnum<class "Telegram Class.lvclass">)  [unwired: 7 in]
            n140 = Index Array(array=w467, index=w462) -> (element=w466:T11)
            n141 = Unbundle By Name(w466) -> ("id"=w463:i64)
            n142 = call-dynamic "Write select user_id.vi"("error in (no error)"=w464, "select user_id"=w463, "Telegram Class in"=w465) -> ("error out"=w472:errorcluster, "Telegram Class out"=w473:refnum<class "Telegram Class.lvclass">)  [unwired: 7 in]
          }
        }
      }
    }
    "error" <- w86
    n143 = case shown="Error" w86 {
      selector: w86 -> [w95 w97]
      tunnel: [w95 w96] -> w85
      frame No Error {
      }
      frame Error {
        n144 = call <vilib>:"Clear Errors.vi"("error in (no error)"=w97) -> ("error out"=w96:errorcluster)  [unwired: 5 in, 1 out]
      }
    }
    n145 = case shown="Default" w87 {
      selector: w87 -> [_ w98]
      frame "" {
      }
      frame Default {
        "JSON" <- w98
      }
    }
  }
  n146 = Unregister For Events(event registration refnum=w12, error in=w11) -> (error out=w1:errorcluster)
  n147 = Merge Errors(w16, w1) -> (w9:errorcluster)
  n148 = Destroy User Event(user event=w10, error in=w9) -> (error out=w7:errorcluster)
  n149 = call <vilib>:"General Error Handler.vi"("error in (no error)"=w7) -> ()  [unwired: 10 in, 5 out]
